vi "sub_SPNs.vi"() -> (0 "SPNs":T1(array[cluster])=[{"SPN"=520192, "Name"="转矩P", "SlotType"=enum."Percent", "Unit"=enum."%", "Value"=variant, "Scaling"=0.4, "LowLmt"=0.0, "HighLmt"=100.0, "Offset"=0.0, "Length"=8, "PGN"=65280, "Comment"="设定转矩的P参数", "LastUpdate"=timestamp(0 s since 1904-01-01)}, {"SPN"=520193, "Name"="转矩I", "SlotType"=enum."Percent", "Unit"=enum."%", "Value"=variant, "Scaling"=0.4, "LowLmt"=0.0, "HighLmt"=100.0, "Offset"=0.0, "Length"=8, "PGN"=65280, "Comment"="设定转矩的I参数", "LastUpdate"=timestamp(0 s since 1904-01-01)}, {"SPN"=520194, "Name"="转矩D", "SlotType"=enum."Percent", "Unit"=enum."%", "Value"=variant, "Scaling"=0.4, "LowLmt"=0.0, "HighLmt"=100.0, "Offset"=0.0, "Length"=8, "PGN"=65280, "Comment"="设定转矩的D参数", "LastUpdate"=timestamp(0 s since 1904-01-01)}, {"SPN"=520195, "Name"="激磁P", "SlotType"=enum."Percent", "Unit"=enum."%", "Value"=variant, "Scaling"=0.4, "LowLmt"=0.0, "HighLmt"=100.0, "Offset"=0.0, "Length"=8, "PGN"=65280, "Comment"="设定激磁的P参数", "LastUpdate"=timestamp(0 s since 1904-01-01)}, {"SPN"=520196, "Name"="激磁I", "SlotType"=enum."Percent", "Unit"=enum."%", "Value"=variant, "Scaling"=0.4, "LowLmt"=0.0, "HighLmt"=100.0, "Offset"=0.0, "Length"=8, "PGN"=65280, "Comment"="设定激磁的I参数", "LastUpdate"=timestamp(0 s since 1904-01-01)}, {"SPN"=520197, "Name"="激磁D", "SlotType"=enum."Percent", "Unit"=enum."%", "Value"=variant, "Scaling"=0.4, "LowLmt"=0.0, "HighLmt"=100.0, "Offset"=0.0, "Length"=8, "PGN"=65280, "Comment"="设定激磁的D参数", "LastUpdate"=timestamp(0 s since 1904-01-01)}, {"SPN"=520198, "Name"="怠速转矩", "SlotType"=enum."Percent", "Unit"=enum."%", "Value"=variant, "Scaling"=0.4, "LowLmt"=0.0, "HighLmt"=100.0, "Offset"=0.0, "Length"=8, "PGN"=65280, "Comment"="", "LastUpdate"=timestamp(0 s since 1904-01-01)}, {"SPN"=520199, "Name"="防滑转矩", "SlotType"=enum."Percent", "Unit"=enum."%", "Value"=variant, "Scaling"=0.4, "LowLmt"=0.0, "HighLmt"=100.0, "Offset"=0.0, "Length"=8, "PGN"=65280, "Comment"="", "LastUpdate"=timestamp(0 s since 1904-01-01)}, {"SPN"=520200, "Name"="滑差", "SlotType"=enum."Number of bytes", "Unit"=enum."1", "Value"=variant, "Scaling"=1.0, "LowLmt"=0.0, "HighLmt"=200.0, "Offset"=0.0, "Length"=8, "PGN"=65280, "Comment"="", "LastUpdate"=timestamp(0 s since 1904-01-01)}, {"SPN"=520201, "Name"="S to RPM", "SlotType"=enum."Velocity, rotational", "Unit"=enum."rpm", "Value"=variant, "Scaling"=0.125, "LowLmt"=0.0, "HighLmt"=8031.875, "Offset"=0.0, "Length"=16, "PGN"=65280, "Comment"="", "LastUpdate"=timestamp(0 s since 1904-01-01)}, {"SPN"=520202, "Name"="弱磁速度", "SlotType"=enum."Velocity, rotational", "Unit"=enum."rpm", "Value"=variant, "Scaling"=0.125, "LowLmt"=0.0, "HighLmt"=8031.875, "Offset"=0.0, "Length"=16, "PGN"=65280, "Comment"="", "LastUpdate"=timestamp(0 s since 1904-01-01)}, {"SPN"=520203, "Name"="D-C限制", "SlotType"=enum."Percent", "Unit"=enum."%", "Value"=variant, "Scaling"=0.4, "LowLmt"=0.0, "HighLmt"=100.0, "Offset"=0.0, "Length"=8, "PGN"=65280, "Comment"="限制控制器的最大驱动电流", "LastUpdate"=timestamp(0 s since 1904-01-01)}, {"SPN"=520204, "Name"="1Delta最大", "SlotType"=enum."Percent", "Unit"=enum."%", "Value"=variant, "Scaling"=0.4, "LowLmt"=0.0, "HighLmt"=100.0, "Offset"=0.0, "Length"=8, "PGN"=65280, "Comment"="限制1倍Delta下的最大功率", "LastUpdate"=timestamp(0 s since 1904-01-01)}, {"SPN"=520205, "Name"="R-C限制", "SlotType"=enum."Percent", "Unit"=enum."%", "Value"=variant, "Scaling"=0.4, "LowLmt"=0.0, "HighLmt"=100.0, "Offset"=0.0, "Length"=8, "PGN"=65280, "Comment"="限制最大回馈电流", "LastUpdate"=timestamp(0 s since 1904-01-01)}, {"SPN"=520206, "Name"="额定转速", "SlotType"=enum."Velocity, rotational", "Unit"=enum."rpm", "Value"=variant, "Scaling"=0.125, "LowLmt"=0.0, "HighLmt"=8031.875, "Offset"=0.0, "Length"=16, "PGN"=65280, "Comment"="", "LastUpdate"=timestamp(0 s since 1904-01-01)}, {"SPN"=520207, "Name"="Delta转速", "SlotType"=enum."Velocity, rotational", "Unit"=enum."rpm", "Value"=variant, "Scaling"=0.125, "LowLmt"=0.0, "HighLmt"=8031.875, "Offset"=0.0, "Length"=16, "PGN"=65280, "Comment"="", "LastUpdate"=timestamp(0 s since 1904-01-01)}, {"SPN"=520208, "Name"="额定最大", "SlotType"=enum."Percent", "Unit"=enum."%", "Value"=variant, "Scaling"=0.4, "LowLmt"=0.0, "HighLmt"=100.0, "Offset"=0.0, "Length"=8, "PGN"=65280, "Comment"="限制额定转速下的最大功率", "LastUpdate"=timestamp(0 s since 1904-01-01)}, {"SPN"=520209, "Name"="2Delta最大", "SlotType"=enum."Percent", "Unit"=enum."%", "Value"=variant, "Scaling"=0.4, "LowLmt"=0.0, "HighLmt"=100.0, "Offset"=0.0, "Length"=8, "PGN"=65280, "Comment"="限制2倍Delta下的最大功率", "LastUpdate"=timestamp(0 s since 1904-01-01)}, {"SPN"=520210, "Name"="4Delta最大", "SlotType"=enum."Percent", "Unit"=enum."%", "Value"=variant, "Scaling"=0.4, "LowLmt"=0.0, "HighLmt"=100.0, "Offset"=0.0, "Length"=8, "PGN"=65280, "Comment"="限制4倍Delta下的最大功率", "LastUpdate"=timestamp(0 s since 1904-01-01)}, {"SPN"=520211, "Name"="8Delta最大", "SlotType"=enum."Percent", "Unit"=enum."%", "Value"=variant, "Scaling"=0.4, "LowLmt"=0.0, "HighLmt"=100.0, "Offset"=0.0, "Length"=8, "PGN"=65280, "Comment"="限制8倍Delta下的最大功率", "LastUpdate"=timestamp(0 s since 1904-01-01)}, {"SPN"=520212, "Name"="ACC Rate", "SlotType"=enum."Time", "Unit"=enum."s", "Value"=variant, "Scaling"=0.1, "LowLmt"=0.0, "HighLmt"=25.0, "Offset"=0.0, "Length"=8, "PGN"=65280, "Comment"="当满踏板的时候,设置转矩从0到最大值的响应时间", "LastUpdate"=timestamp(0 s since 1904-01-01)}, {"SPN"=520213, "Name"="ACC R-Rate", "SlotType"=enum."Time", "Unit"=enum."s", "Value"=variant, "Scaling"=0.1, "LowLmt"=0.0, "HighLmt"=25.0, "Offset"=0.0, "Length"=8, "PGN"=65280, "Comment"="当汽车还在加速的时候,松掉加速踏板后,设置开始减速的时间", "LastUpdate"=timestamp(0 s since 1904-01-01)}, {"SPN"=520214, "Name"="B Rate", "SlotType"=enum."Time", "Unit"=enum."s", "Value"=variant, "Scaling"=0.1, "LowLmt"=0.0, "HighLmt"=25.0, "Offset"=0.0, "Length"=8, "PGN"=65280, "Comment"="当汽车还在行使时,踩下刹车踏板后,设置制动转矩开始的时间", "LastUpdate"=timestamp(0 s since 1904-01-01)}, {"SPN"=520215, "Name"="B R-Rate", "SlotType"=enum."Time", "Unit"=enum."s", "Value"=variant, "Scaling"=0.1, "LowLmt"=0.0, "HighLmt"=25.0, "Offset"=0.0, "Length"=8, "PGN"=65280, "Comment"="当汽车在刹车过程中,松掉刹车踏板后,设置制动转矩释放的时间", "LastUpdate"=timestamp(0 s since 1904-01-01)}, {"SPN"=520216, "Name"="加速Min", "SlotType"=enum."Electrical Voltage", "Unit"=enum."V", "Value"=variant, "Scaling"=0.01, "LowLmt"=0.0, "HighLmt"=642.55, "Offset"=0.0, "Length"=16, "PGN"=65280, "Comment"="设置加速踏板的最小电压", "LastUpdate"=timestamp(0 s since 1904-01-01)}, {"SPN"=520217, "Name"="加速Max", "SlotType"=enum."Electrical Voltage", "Unit"=enum."V", "Value"=variant, "Scaling"=0.01, "LowLmt"=0.0, "HighLmt"=642.55, "Offset"=0.0, "Length"=16, "PGN"=65280, "Comment"="设置加速踏板的最大电压", "LastUpdate"=timestamp(0 s since 1904-01-01)}, {"SPN"=520218, "Name"="刹车Min", "SlotType"=enum."Electrical Voltage", "Unit"=enum."V", "Value"=variant, "Scaling"=0.01, "LowLmt"=0.0, "HighLmt"=642.55, "Offset"=0.0, "Length"=16, "PGN"=65280, "Comment"="设置刹车踏板的最小电压", "LastUpdate"=timestamp(0 s since 1904-01-01)}, {"SPN"=520219, "Name"="加速Map", "SlotType"=enum."Percent", "Unit"=enum."%", "Value"=variant, "Scaling"=0.4, "LowLmt"=0.0, "HighLmt"=100.0, "Offset"=0.0, "Length"=8, "PGN"=65280, "Comment"="设置加速踏板对应的加速曲线", "LastUpdate"=timestamp(0 s since 1904-01-01)}, {"SPN"=520220, "Name"="刹车Max", "SlotType"=enum."Electrical Voltage", "Unit"=enum."V", "Value"=variant, "Scaling"=0.01, "LowLmt"=0.0, "HighLmt"=642.55, "Offset"=0.0, "Length"=16, "PGN"=65280, "Comment"="设置刹车踏板的最大电压", "LastUpdate"=timestamp(0 s since 1904-01-01)}, {"SPN"=520221, "Name"="刹车Map", "SlotType"=enum."Percent", "Unit"=enum."%", "Value"=variant, "Scaling"=0.4, "LowLmt"=0.0, "HighLmt"=100.0, "Offset"=0.0, "Length"=8, "PGN"=65280, "Comment"="设置刹车踏板对应的刹车曲线", "LastUpdate"=timestamp(0 s since 1904-01-01)}, {"SPN"=520256, "Name"="远程加速踏板给定", "SlotType"=enum."Percent", "Unit"=enum."%", "Value"=variant, "Scaling"=0.4, "LowLmt"=0.0, "HighLmt"=100.0, "Offset"=0.0, "Length"=8, "PGN"=65281, "Comment"="远程加速踏板给定值", "LastUpdate"=timestamp(0 s since 1904-01-01)}, {"SPN"=520257, "Name"="远程刹车踏板给定", "SlotType"=enum."Percent", "Unit"=enum."%", "Value"=variant, "Scaling"=0.4, "LowLmt"=0.0, "HighLmt"=100.0, "Offset"=0.0, "Length"=8, "PGN"=65281, "Comment"="远程刹车踏板给定值", "LastUpdate"=timestamp(0 s since 1904-01-01)}, {"SPN"=520258, "Name"="远程档位给定", "SlotType"=enum."Bit Field", "Unit"=enum."1", "Value"=variant, "Scaling"=0.0, "LowLmt"=0.0, "HighLmt"=250.0, "Offset"=0.0, "Length"=8, "PGN"=65281, "Comment"="1:P,2:N,3:D,4:R", "LastUpdate"=timestamp(0 s since 1904-01-01)}, {"SPN"=520259, "Name"="远程调试模式使能", "SlotType"=enum."Bool", "Unit"=enum."bit", "Value"=variant, "Scaling"=0.0, "LowLmt"=0.0, "HighLmt"=1.0, "Offset"=0.0, "Length"=1, "PGN"=65281, "Comment"="远程调试模式开关", "LastUpdate"=timestamp(0 s since 1904-01-01)}, {"SPN"=520260, "Name"="远程加速踏板给定使能", "SlotType"=enum."Bool", "Unit"=enum."bit", "Value"=variant, "Scaling"=0.0, "LowLmt"=0.0, "HighLmt"=1.0, "Offset"=0.0, "Length"=1, "PGN"=65281, "Comment"="远程加速踏板给定开关，远程调试模式开关=T时有效", "LastUpdate"=timestamp(0 s since 1904-01-01)}, {"SPN"=520261, "Name"="远程刹车踏板给定使能", "SlotType"=enum."Bool", "Unit"=enum."bit", "Value"=variant, "Scaling"=0.0, "LowLmt"=0.0, "HighLmt"=1.0, "Offset"=0.0, "Length"=1, "PGN"=65281, "Comment"="远程刹车踏板给定开关，远程调试模式开关=T时有效", "LastUpdate"=timestamp(0 s since 1904-01-01)}, {"SPN"=520262, "Name"="远程档位给定使能", "SlotType"=enum."Bool", "Unit"=enum."bit", "Value"=variant, "Scaling"=0.0, "LowLmt"=0.0, "HighLmt"=1.0, "Offset"=0.0, "Length"=1, "PGN"=65281, "Comment"="远程档位给定开关，远程调试模式开关=T时有效", "LastUpdate"=timestamp(0 s since 1904-01-01)}, {"SPN"=520266, "Name"="给定电压", "SlotType"=enum."Percent", "Unit"=enum."%", "Value"=variant, "Scaling"=0.002, "LowLmt"=0.0, "HighLmt"=100.0, "Offset"=0.0, "Length"=16, "PGN"=65282, "Comment"="压频模式给定电压百分比", "LastUpdate"=timestamp(0 s since 1904-01-01)}, {"SPN"=520267, "Name"="给定频率", "SlotType"=enum."Percent", "Unit"=enum."%", "Value"=variant, "Scaling"=0.002, "LowLmt"=0.0, "HighLmt"=100.0, "Offset"=0.0, "Length"=16, "PGN"=65282, "Comment"="压频模式给定频率百分比", "LastUpdate"=timestamp(0 s since 1904-01-01)}, {"SPN"=520268, "Name"="给定电压使能", "SlotType"=enum."Bool", "Unit"=enum."bit", "Value"=variant, "Scaling"=0.0, "LowLmt"=0.0, "HighLmt"=1.0, "Offset"=0.0, "Length"=1, "PGN"=65282, "Comment"="是否允许通过通信方式给定电压", "LastUpdate"=timestamp(0 s since 1904-01-01)}, {"SPN"=520269, "Name"="给定频率使能", "SlotType"=enum."Bool", "Unit"=enum."bit", "Value"=variant, "Scaling"=0.0, "LowLmt"=0.0, "HighLmt"=1.0, "Offset"=0.0, "Length"=1, "PGN"=65282, "Comment"="是否允许通过通信方式给定频率", "LastUpdate"=timestamp(0 s since 1904-01-01)}, {"SPN"=520272, "Name"="电机转速", "SlotType"=enum."Velocity, rotational", "Unit"=enum."rpm", "Value"=variant, "Scaling"=0.153, "LowLmt"=0.0, "HighLmt"=10000.0, "Offset"=0.0, "Length"=16, "PGN"=65290, "Comment"="电机的转速", "LastUpdate"=timestamp(0 s since 1904-01-01)}, {"SPN"=520273, "Name"="控制器温度", "SlotType"=enum."Temperature", "Unit"=enum."℃", "Value"=variant, "Scaling"=0.03125, "LowLmt"=-273.0, "HighLmt"=1735.0, "Offset"=-273.0, "Length"=16, "PGN"=65290, "Comment"="控制器实际温度", "LastUpdate"=timestamp(0 s since 1904-01-01)}, {"SPN"=520274, "Name"="电机温度", "SlotType"=enum."Temperature", "Unit"=enum."℃", "Value"=variant, "Scaling"=0.03125, "LowLmt"=-273.0, "HighLmt"=1735.0, "Offset"=-273.0, "Length"=16, "PGN"=65290, "Comment"="电机的实际温度", "LastUpdate"=timestamp(0 s since 1904-01-01)}, {"SPN"=520275, "Name"="控制器过压", "SlotType"=enum."Bool", "Unit"=enum."bit", "Value"=variant, "Scaling"=1.0, "LowLmt"=0.0, "HighLmt"=1.0, "Offset"=0.0, "Length"=1, "PGN"=65290, "Comment"="指示控制器是否过压", "LastUpdate"=timestamp(0 s since 1904-01-01)}, {"SPN"=520276, "Name"="控制器欠压", "SlotType"=enum."Bool", "Unit"=enum."bit", "Value"=variant, "Scaling"=1.0, "LowLmt"=0.0, "HighLmt"=1.0, "Offset"=0.0, "Length"=1, "PGN"=65290, "Comment"="指示控制器是否欠压", "LastUpdate"=timestamp(0 s since 1904-01-01)}, {"SPN"=520277, "Name"="控制器过流", "SlotType"=enum."Bool", "Unit"=enum."bit", "Value"=variant, "Scaling"=1.0, "LowLmt"=0.0, "HighLmt"=1.0, "Offset"=0.0, "Length"=1, "PGN"=65290, "Comment"="指示控制器是否过流", "LastUpdate"=timestamp(0 s since 1904-01-01)}, {"SPN"=520278, "Name"="控制器过温", "SlotType"=enum."Bool", "Unit"=enum."bit", "Value"=variant, "Scaling"=1.0, "LowLmt"=0.0, "HighLmt"=1.0, "Offset"=0.0, "Length"=1, "PGN"=65290, "Comment"="指示控制器是否过温", "LastUpdate"=timestamp(0 s since 1904-01-01)}, {"SPN"=520279, "Name"="控制器保护", "SlotType"=enum."Bool", "Unit"=enum."bit", "Value"=variant, "Scaling"=1.0, "LowLmt"=0.0, "HighLmt"=1.0, "Offset"=0.0, "Length"=1, "PGN"=65290, "Comment"="指示控制器是否保护", "LastUpdate"=timestamp(0 s since 1904-01-01)}, {"SPN"=520280, "Name"="其他故障", "SlotType"=enum."Bool", "Unit"=enum."bit", "Value"=variant, "Scaling"=1.0, "LowLmt"=0.0, "HighLmt"=1.0, "Offset"=0.0, "Length"=1, "PGN"=65290, "Comment"="指示控制器是否发生其他故障", "LastUpdate"=timestamp(0 s since 1904-01-01)}, {"SPN"=520281, "Name"="母线电流", "SlotType"=enum."Electrical Current", "Unit"=enum."A", "Value"=variant, "Scaling"=0.05, "LowLmt"=-1600.0, "HighLmt"=1612.75, "Offset"=-1600.0, "Length"=16, "PGN"=65290, "Comment"="电池组母线电流", "LastUpdate"=timestamp(0 s since 1904-01-01)}, {"SPN"=520288, "Name"="母线电压", "SlotType"=enum."Electrical Voltage", "Unit"=enum."V", "Value"=variant, "Scaling"=0.01, "LowLmt"=0.0, "HighLmt"=642.55, "Offset"=0.0, "Length"=16, "PGN"=65291, "Comment"="电池组母线电压", "LastUpdate"=timestamp(0 s since 1904-01-01)}, {"SPN"=520289, "Name"="电机电压", "SlotType"=enum."Electrical Voltage", "Unit"=enum."V", "Value"=variant, "Scaling"=0.01, "LowLmt"=0.0, "HighLmt"=642.55, "Offset"=0.0, "Length"=16, "PGN"=65291, "Comment"="电机端电压有效值", "LastUpdate"=timestamp(0 s since 1904-01-01)}, {"SPN"=520290, "Name"="电机电流", "SlotType"=enum."Electrical Current", "Unit"=enum."A", "Value"=variant, "Scaling"=0.05, "LowLmt"=-1600.0, "HighLmt"=1612.75, "Offset"=-1600.0, "Length"=16, "PGN"=65291, "Comment"="电机端电流有效值", "LastUpdate"=timestamp(0 s since 1904-01-01)}, {"SPN"=520291, "Name"="档位", "SlotType"=enum."Bit Field", "Unit"=enum."1", "Value"=variant, "Scaling"=1.0, "LowLmt"=0.0, "HighLmt"=250.0, "Offset"=0.0, "Length"=4, "PGN"=65291, "Comment"="1:P,2:N,3:D,4:R", "LastUpdate"=timestamp(0 s since 1904-01-01)}, {"SPN"=520292, "Name"="加速给定", "SlotType"=enum."Percent", "Unit"=enum."%", "Value"=variant, "Scaling"=0.4, "LowLmt"=0.0, "HighLmt"=100.0, "Offset"=0.0, "Length"=8, "PGN"=65291, "Comment"="加速踏板百分比", "LastUpdate"=timestamp(0 s since 1904-01-01)}, {"SPN"=520293, "Name"="刹车给定", "SlotType"=enum."Percent", "Unit"=enum."%", "Value"=variant, "Scaling"=0.4, "LowLmt"=0.0, "HighLmt"=100.0, "Offset"=0.0, "Length"=8, "PGN"=65291, "Comment"="刹车踏板百分比", "LastUpdate"=timestamp(0 s since 1904-01-01)}, {"SPN"=520294, "Name"="频率", "SlotType"=enum."Frequency", "Unit"=enum."Hz", "Value"=variant, "Scaling"=0.0078125, "LowLmt"=0.0, "HighLmt"=501.9921875, "Offset"=0.0, "Length"=16, "PGN"=65291, "Comment"="电机同步频率", "LastUpdate"=timestamp(0 s since 1904-01-01)}, {"SPN"=520295, "Name"="直流功率", "SlotType"=enum."Power, Real", "Unit"=enum."kW", "Value"=variant, "Scaling"=0.002, "LowLmt"=0.0, "HighLmt"=128.51, "Offset"=0.0, "Length"=16, "PGN"=65291, "Comment"="控制器直流母线输入功率", "LastUpdate"=timestamp(0 s since 1904-01-01)}, {"SPN"=520296, "Name"="加速开关", "SlotType"=enum."Bool", "Unit"=enum."bit", "Value"=variant, "Scaling"=1.0, "LowLmt"=0.0, "HighLmt"=1.0, "Offset"=0.0, "Length"=1, "PGN"=65291, "Comment"="指示汽车加速踏板是否塌下", "LastUpdate"=timestamp(0 s since 1904-01-01)}, {"SPN"=520297, "Name"="刹车开关", "SlotType"=enum."Bool", "Unit"=enum."bit", "Value"=variant, "Scaling"=1.0, "LowLmt"=0.0, "HighLmt"=1.0, "Offset"=0.0, "Length"=1, "PGN"=65291, "Comment"="指示汽车刹车踏板是否塌下", "LastUpdate"=timestamp(0 s since 1904-01-01)}, {"SPN"=520298, "Name"="座椅开关", "SlotType"=enum."Bool", "Unit"=enum."bit", "Value"=variant, "Scaling"=1.0, "LowLmt"=0.0, "HighLmt"=1.0, "Offset"=0.0, "Length"=1, "PGN"=65291, "Comment"="指示汽车驾驶员座椅是否处于坐姿状态", "LastUpdate"=timestamp(0 s since 1904-01-01)}, {"SPN"=520299, "Name"="电机正转", "SlotType"=enum."Bool", "Unit"=enum."bit", "Value"=variant, "Scaling"=1.0, "LowLmt"=0.0, "HighLmt"=1.0, "Offset"=0.0, "Length"=1, "PGN"=65291, "Comment"="电机正转还是反转", "LastUpdate"=timestamp(0 s since 1904-01-01)}, {"SPN"=520304, "Name"="母线电压", "SlotType"=enum."Electrical Voltage", "Unit"=enum."V", "Value"=variant, "Scaling"=0.01, "LowLmt"=0.0, "HighLmt"=642.55, "Offset"=0.0, "Length"=16, "PGN"=65292, "Comment"="电池组母线电压", "LastUpdate"=timestamp(0 s since 1904-01-01)}, {"SPN"=520305, "Name"="电机电压", "SlotType"=enum."Electrical Voltage", "Unit"=enum."V", "Value"=variant, "Scaling"=0.01, "LowLmt"=0.0, "HighLmt"=642.55, "Offset"=0.0, "Length"=16, "PGN"=65292, "Comment"="电机端电压有效值", "LastUpdate"=timestamp(0 s since 1904-01-01)}, {"SPN"=520306, "Name"="给定电压", "SlotType"=enum."Electrical Voltage", "Unit"=enum."%", "Value"=variant, "Scaling"=0.01, "LowLmt"=0.0, "HighLmt"=642.55, "Offset"=0.0, "Length"=16, "PGN"=65292, "Comment"="给定电压百分比", "LastUpdate"=timestamp(0 s since 1904-01-01)}, {"SPN"=520307, "Name"="效率", "SlotType"=enum."Percent", "Unit"=enum."%", "Value"=variant, "Scaling"=0.4, "LowLmt"=0.0, "HighLmt"=100.0, "Offset"=0.0, "Length"=8, "PGN"=65292, "Comment"="控制器效率", "LastUpdate"=timestamp(0 s since 1904-01-01)}, {"SPN"=520308, "Name"="U相电流", "SlotType"=enum."Electrical Current", "Unit"=enum."A", "Value"=variant, "Scaling"=0.05, "LowLmt"=-1600.0, "HighLmt"=1612.75, "Offset"=-1600.0, "Length"=16, "PGN"=65292, "Comment"="电机U相电流有效值", "LastUpdate"=timestamp(0 s since 1904-01-01)}, {"SPN"=520309, "Name"="V相电流", "SlotType"=enum."Electrical Current", "Unit"=enum."A", "Value"=variant, "Scaling"=0.05, "LowLmt"=-1600.0, "HighLmt"=1612.75, "Offset"=-1600.0, "Length"=16, "PGN"=65292, "Comment"="电机V相电流有效值", "LastUpdate"=timestamp(0 s since 1904-01-01)}, {"SPN"=520310, "Name"="W相电流", "SlotType"=enum."Electrical Current", "Unit"=enum."A", "Value"=variant, "Scaling"=0.05, "LowLmt"=-1600.0, "HighLmt"=1612.75, "Offset"=-1600.0, "Length"=16, "PGN"=65292, "Comment"="电机W相电流有效值", "LastUpdate"=timestamp(0 s since 1904-01-01)}, {"SPN"=520311, "Name"="电机正转", "SlotType"=enum."Bool", "Unit"=enum."bit", "Value"=variant, "Scaling"=1.0, "LowLmt"=0.0, "HighLmt"=1.0, "Offset"=0.0, "Length"=1, "PGN"=65292, "Comment"="电机正转还是反转", "LastUpdate"=timestamp(0 s since 1904-01-01)}, {"SPN"=520312, "Name"="后退", "SlotType"=enum."Bool", "Unit"=enum."bit", "Value"=variant, "Scaling"=1.0, "LowLmt"=0.0, "HighLmt"=1.0, "Offset"=0.0, "Length"=1, "PGN"=65292, "Comment"="是否倒档", "LastUpdate"=timestamp(0 s since 1904-01-01)}, {"SPN"=520313, "Name"="前进", "SlotType"=enum."Bool", "Unit"=enum."bit", "Value"=variant, "Scaling"=1.0, "LowLmt"=0.0, "HighLmt"=1.0, "Offset"=0.0, "Length"=1, "PGN"=65292, "Comment"="是否前进档", "LastUpdate"=timestamp(0 s since 1904-01-01)}, {"SPN"=520314, "Name"="加速踏板", "SlotType"=enum."Bool", "Unit"=enum."bit", "Value"=variant, "Scaling"=1.0, "LowLmt"=0.0, "HighLmt"=1.0, "Offset"=0.0, "Length"=1, "PGN"=65292, "Comment"="加速踏板已踏下", "LastUpdate"=timestamp(0 s since 1904-01-01)}, {"SPN"=520315, "Name"="刹车踏板", "SlotType"=enum."Bool", "Unit"=enum."bit", "Value"=variant, "Scaling"=1.0, "LowLmt"=0.0, "HighLmt"=1.0, "Offset"=0.0, "Length"=1, "PGN"=65292, "Comment"="刹车踏板已踏下", "LastUpdate"=timestamp(0 s since 1904-01-01)}, {"SPN"=520316, "Name"="巡航开关", "SlotType"=enum."Bool", "Unit"=enum."bit", "Value"=variant, "Scaling"=1.0, "LowLmt"=0.0, "HighLmt"=1.0, "Offset"=0.0, "Length"=1, "PGN"=65292, "Comment"="巡航功能开启", "LastUpdate"=timestamp(0 s since 1904-01-01)}, {"SPN"=520317, "Name"="座椅开关", "SlotType"=enum."Bool", "Unit"=enum."bit", "Value"=variant, "Scaling"=1.0, "LowLmt"=0.0, "HighLmt"=1.0, "Offset"=0.0, "Length"=1, "PGN"=65292, "Comment"="座椅开关", "LastUpdate"=timestamp(0 s since 1904-01-01)}, {"SPN"=520318, "Name"="给定频率", "SlotType"=enum."Frequency", "Unit"=enum."Hz", "Value"=variant, "Scaling"=0.0078125, "LowLmt"=0.0, "HighLmt"=501.9921875, "Offset"=0.0, "Length"=16, "PGN"=65292, "Comment"="给定频率值", "LastUpdate"=timestamp(0 s since 1904-01-01)}, {"SPN"=520319, "Name"="频率", "SlotType"=enum."Frequency", "Unit"=enum."Hz", "Value"=variant, "Scaling"=0.0078125, "LowLmt"=0.0, "HighLmt"=501.9921875, "Offset"=0.0, "Length"=16, "PGN"=65292, "Comment"="电机同步频率值", "LastUpdate"=timestamp(0 s since 1904-01-01)}, {"SPN"=520320, "Name"="转差频率", "SlotType"=enum."Frequency", "Unit"=enum."Hz", "Value"=variant, "Scaling"=0.0078125, "LowLmt"=0.0, "HighLmt"=501.9921875, "Offset"=0.0, "Length"=16, "PGN"=65292, "Comment"="转差频率值", "LastUpdate"=timestamp(0 s since 1904-01-01)}, {"SPN"=520321, "Name"="直流功率", "SlotType"=enum."Power, Real", "Unit"=enum."kW", "Value"=variant, "Scaling"=0.002, "LowLmt"=0.0, "HighLmt"=128.51, "Offset"=0.0, "Length"=16, "PGN"=65292, "Comment"="控制器直流母线输入功率", "LastUpdate"=timestamp(0 s since 1904-01-01)}, {"SPN"=520322, "Name"="输出功率", "SlotType"=enum."Power, Real", "Unit"=enum."kW", "Value"=variant, "Scaling"=0.002, "LowLmt"=0.0, "HighLmt"=128.51, "Offset"=0.0, "Length"=16, "PGN"=65292, "Comment"="控制器输出功率", "LastUpdate"=timestamp(0 s since 1904-01-01)}, {"SPN"=520323, "Name"="输出转矩", "SlotType"=enum."Torque", "Unit"=enum."Nm", "Value"=variant, "Scaling"=0.01, "LowLmt"=-320.0, "HighLmt"=322.55, "Offset"=-320.0, "Length"=16, "PGN"=65292, "Comment"="输出转矩值", "LastUpdate"=timestamp(0 s since 1904-01-01)}, {"SPN"=520324, "Name"="给定转速", "SlotType"=enum."Velocity, rotational", "Unit"=enum."rpm", "Value"=variant, "Scaling"=0.125, "LowLmt"=0.0, "HighLmt"=8031.875, "Offset"=0.0, "Length"=16, "PGN"=65292, "Comment"="电机的给定转速", "LastUpdate"=timestamp(0 s since 1904-01-01)}, {"SPN"=520325, "Name"="转差转速", "SlotType"=enum."Velocity, rotational", "Unit"=enum."rpm", "Value"=variant, "Scaling"=0.125, "LowLmt"=0.0, "HighLmt"=8031.875, "Offset"=0.0, "Length"=16, "PGN"=65292, "Comment"="电机的转差转速", "LastUpdate"=timestamp(0 s since 1904-01-01)}, {"SPN"=520326, "Name"="给定电压百分比", "SlotType"=enum."Percent", "Unit"=enum."%", "Value"=variant, "Scaling"=0.01, "LowLmt"=0.0, "HighLmt"=100.0, "Offset"=0.0, "Length"=16, "PGN"=65292, "Comment"="给定电压与母线电压的比值×100%", "LastUpdate"=timestamp(0 s since 1904-01-01)}] {"LastUpdate" format="%<%.3X>T"})   [LabVIEW 2011]
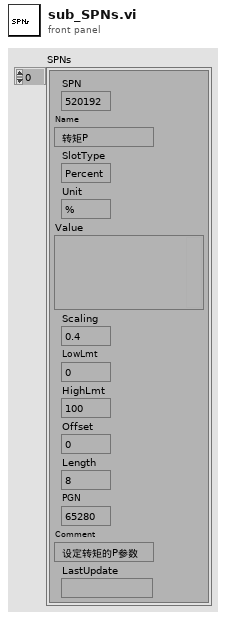
[diagram p1: front panel]
types:
  T1 = cluster{"SPN":u32, "Name":string, "SlotType":enum16{"Unknown Type", "Acceleration", "Angle", "ASCII", "Bool", "Brake Applications", "Bit Field", "Number of bytes", "Capacity, Battery", "Control byte", "Calendar, days", "Calendar, months", "Conductivity", "Count", "Calendar, weeks", "Calendar, years", "Dielectricity", "Direction", "Distance", "Electrical Current", "Economy, gaseous", "Economy, liquid", "Energy", "Electrical Voltage", "Flow rate, gaseous", "Flow rate, liquid", "FMI", "Frequency", "Force", "Fuel Used,gaseous", "Fuel Used, liquid", "Flow rate,volumetric", "Group Function", "Governor gain", "Gear Ratio", "Gear Value", "Identifier", "Inertia", "Intensity, optical", "Kinematic viscosity", "level", "Mass,cargo", "Name (short)", "Name (long)", "OC", "Power, Apparent", "Percent", "Percent,concentration", "Proprietary Data", "position", "Power Factor", "Parts Per Million", "Pressure", "Pressure Rate Change", "Power, Reactive", "Power, Real", "Ratio", "Road Curvature", "Record", "Revolutions", "Source Address", "Specific Gravity", "SPN", "Specific Resistance", "Step", "Transfer Data", "Time", "Temperature", "Torque", "Velocity,angular", "VariantData", "Velocity, linear", "Velocity, magnitude", "Volume", "Velocity, rotational"}, "Unit":enum16{"UnDefined", "%", "1", "1/km", "A", "ASCII", "bin", "bit", "℃", "D", "deg", "deg/s", "g", "Hz", "ID", "kg", "kg/h", "kg/m^2", "km", "km/kg", "km/L", "kPa", "kph", "kW", "kWh", "L", "L/h", "m", "m/h", "m/s", "m/s^2", "m^3/h", "mAh", "min", "mm", "mm^2/s", "Mon", "ms", "mSi/mm", "mW/cm^2", "N", "Nm", "Pa/s", "ppm", "r", "rad/s", "Rat", "Rec", "rpm", "s", "SA", "step", "TF", "V", "VA", "VAr", "W", "Y", "Ωm"}, "Value":variant, "Scaling":dbl, "LowLmt":dbl, "HighLmt":dbl, "Offset":dbl, "Length":u8, "PGN":u32, "Comment":string, "LastUpdate":timestamp}[]
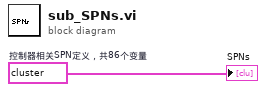
[diagram p0: block diagram]
diagram:
  w1 = T1 [{"SPN"=520192, "Name"="转矩P", "SlotType"=enum."Percent", "Unit"=enum."%", "Value"=variant, "Scaling"=0.4, "LowLmt"=0.0, "HighLmt"=100.0, "Offset"=0.0, "Length"=8, "PGN"=65280, "Comment"="设定转矩的P参数", "LastUpdate"=timestamp(0 s since 1904-01-01)}, {"SPN"=520193, "Name"="转矩I", "SlotType"=enum."Percent", "Unit"=enum."%", "Value"=variant, "Scaling"=0.4, "LowLmt"=0.0, "HighLmt"=100.0, "Offset"=0.0, "Length"=8, "PGN"=65280, "Comment"="设定转矩的I参数", "LastUpdate"=timestamp(0 s since 1904-01-01)}, {"SPN"=520194, "Name"="转矩D", "SlotType"=enum."Percent", "Unit"=enum."%", "Value"=variant, "Scaling"=0.4, "LowLmt"=0.0, "HighLmt"=100.0, "Offset"=0.0, "Length"=8, "PGN"=65280, "Comment"="设定转矩的D参数", "LastUpdate"=timestamp(0 s since 1904-01-01)}, {"SPN"=520195, "Name"="激磁P", "SlotType"=enum."Percent", "Unit"=enum."%", "Value"=variant, "Scaling"=0.4, "LowLmt"=0.0, "HighLmt"=100.0, "Offset"=0.0, "Length"=8, "PGN"=65280, "Comment"="设定激磁的P参数", "LastUpdate"=timestamp(0 s since 1904-01-01)}, {"SPN"=520196, "Name"="激磁I", "SlotType"=enum."Percent", "Unit"=enum."%", "Value"=variant, "Scaling"=0.4, "LowLmt"=0.0, "HighLmt"=100.0, "Offset"=0.0, "Length"=8, "PGN"=65280, "Comment"="设定激磁的I参数", "LastUpdate"=timestamp(0 s since 1904-01-01)}, {"SPN"=520197, "Name"="激磁D", "SlotType"=enum."Percent", "Unit"=enum."%", "Value"=variant, "Scaling"=0.4, "LowLmt"=0.0, "HighLmt"=100.0, "Offset"=0.0, "Length"=8, "PGN"=65280, "Comment"="设定激磁的D参数", "LastUpdate"=timestamp(0 s since 1904-01-01)}, {"SPN"=520198, "Name"="怠速转矩", "SlotType"=enum."Percent", "Unit"=enum."%", "Value"=variant, "Scaling"=0.4, "LowLmt"=0.0, "HighLmt"=100.0, "Offset"=0.0, "Length"=8, "PGN"=65280, "Comment"="", "LastUpdate"=timestamp(0 s since 1904-01-01)}, {"SPN"=520199, "Name"="防滑转矩", "SlotType"=enum."Percent", "Unit"=enum."%", "Value"=variant, "Scaling"=0.4, "LowLmt"=0.0, "HighLmt"=100.0, "Offset"=0.0, "Length"=8, "PGN"=65280, "Comment"="", "LastUpdate"=timestamp(0 s since 1904-01-01)}, {"SPN"=520200, "Name"="滑差", "SlotType"=enum."Number of bytes", "Unit"=enum."1", "Value"=variant, "Scaling"=1.0, "LowLmt"=0.0, "HighLmt"=200.0, "Offset"=0.0, "Length"=8, "PGN"=65280, "Comment"="", "LastUpdate"=timestamp(0 s since 1904-01-01)}, {"SPN"=520201, "Name"="S to RPM", "SlotType"=enum."Velocity, rotational", "Unit"=enum."rpm", "Value"=variant, "Scaling"=0.125, "LowLmt"=0.0, "HighLmt"=8031.875, "Offset"=0.0, "Length"=16, "PGN"=65280, "Comment"="", "LastUpdate"=timestamp(0 s since 1904-01-01)}, {"SPN"=520202, "Name"="弱磁速度", "SlotType"=enum."Velocity, rotational", "Unit"=enum."rpm", "Value"=variant, "Scaling"=0.125, "LowLmt"=0.0, "HighLmt"=8031.875, "Offset"=0.0, "Length"=16, "PGN"=65280, "Comment"="", "LastUpdate"=timestamp(0 s since 1904-01-01)}, {"SPN"=520203, "Name"="D-C限制", "SlotType"=enum."Percent", "Unit"=enum."%", "Value"=variant, "Scaling"=0.4, "LowLmt"=0.0, "HighLmt"=100.0, "Offset"=0.0, "Length"=8, "PGN"=65280, "Comment"="限制控制器的最大驱动电流", "LastUpdate"=timestamp(0 s since 1904-01-01)}, {"SPN"=520204, "Name"="1Delta最大", "SlotType"=enum."Percent", "Unit"=enum."%", "Value"=variant, "Scaling"=0.4, "LowLmt"=0.0, "HighLmt"=100.0, "Offset"=0.0, "Length"=8, "PGN"=65280, "Comment"="限制1倍Delta下的最大功率", "LastUpdate"=timestamp(0 s since 1904-01-01)}, {"SPN"=520205, "Name"="R-C限制", "SlotType"=enum."Percent", "Unit"=enum."%", "Value"=variant, "Scaling"=0.4, "LowLmt"=0.0, "HighLmt"=100.0, "Offset"=0.0, "Length"=8, "PGN"=65280, "Comment"="限制最大回馈电流", "LastUpdate"=timestamp(0 s since 1904-01-01)}, {"SPN"=520206, "Name"="额定转速", "SlotType"=enum."Velocity, rotational", "Unit"=enum."rpm", "Value"=variant, "Scaling"=0.125, "LowLmt"=0.0, "HighLmt"=8031.875, "Offset"=0.0, "Length"=16, "PGN"=65280, "Comment"="", "LastUpdate"=timestamp(0 s since 1904-01-01)}, {"SPN"=520207, "Name"="Delta转速", "SlotType"=enum."Velocity, rotational", "Unit"=enum."rpm", "Value"=variant, "Scaling"=0.125, "LowLmt"=0.0, "HighLmt"=8031.875, "Offset"=0.0, "Length"=16, "PGN"=65280, "Comment"="", "LastUpdate"=timestamp(0 s since 1904-01-01)}, {"SPN"=520208, "Name"="额定最大", "SlotType"=enum."Percent", "Unit"=enum."%", "Value"=variant, "Scaling"=0.4, "LowLmt"=0.0, "HighLmt"=100.0, "Offset"=0.0, "Length"=8, "PGN"=65280, "Comment"="限制额定转速下的最大功率", "LastUpdate"=timestamp(0 s since 1904-01-01)}, {"SPN"=520209, "Name"="2Delta最大", "SlotType"=enum."Percent", "Unit"=enum."%", "Value"=variant, "Scaling"=0.4, "LowLmt"=0.0, "HighLmt"=100.0, "Offset"=0.0, "Length"=8, "PGN"=65280, "Comment"="限制2倍Delta下的最大功率", "LastUpdate"=timestamp(0 s since 1904-01-01)}, {"SPN"=520210, "Name"="4Delta最大", "SlotType"=enum."Percent", "Unit"=enum."%", "Value"=variant, "Scaling"=0.4, "LowLmt"=0.0, "HighLmt"=100.0, "Offset"=0.0, "Length"=8, "PGN"=65280, "Comment"="限制4倍Delta下的最大功率", "LastUpdate"=timestamp(0 s since 1904-01-01)}, {"SPN"=520211, "Name"="8Delta最大", "SlotType"=enum."Percent", "Unit"=enum."%", "Value"=variant, "Scaling"=0.4, "LowLmt"=0.0, "HighLmt"=100.0, "Offset"=0.0, "Length"=8, "PGN"=65280, "Comment"="限制8倍Delta下的最大功率", "LastUpdate"=timestamp(0 s since 1904-01-01)}, {"SPN"=520212, "Name"="ACC Rate", "SlotType"=enum."Time", "Unit"=enum."s", "Value"=variant, "Scaling"=0.1, "LowLmt"=0.0, "HighLmt"=25.0, "Offset"=0.0, "Length"=8, "PGN"=65280, "Comment"="当满踏板的时候,设置转矩从0到最大值的响应时间", "LastUpdate"=timestamp(0 s since 1904-01-01)}, {"SPN"=520213, "Name"="ACC R-Rate", "SlotType"=enum."Time", "Unit"=enum."s", "Value"=variant, "Scaling"=0.1, "LowLmt"=0.0, "HighLmt"=25.0, "Offset"=0.0, "Length"=8, "PGN"=65280, "Comment"="当汽车还在加速的时候,松掉加速踏板后,设置开始减速的时间", "LastUpdate"=timestamp(0 s since 1904-01-01)}, {"SPN"=520214, "Name"="B Rate", "SlotType"=enum."Time", "Unit"=enum."s", "Value"=variant, "Scaling"=0.1, "LowLmt"=0.0, "HighLmt"=25.0, "Offset"=0.0, "Length"=8, "PGN"=65280, "Comment"="当汽车还在行使时,踩下刹车踏板后,设置制动转矩开始的时间", "LastUpdate"=timestamp(0 s since 1904-01-01)}, {"SPN"=520215, "Name"="B R-Rate", "SlotType"=enum."Time", "Unit"=enum."s", "Value"=variant, "Scaling"=0.1, "LowLmt"=0.0, "HighLmt"=25.0, "Offset"=0.0, "Length"=8, "PGN"=65280, "Comment"="当汽车在刹车过程中,松掉刹车踏板后,设置制动转矩释放的时间", "LastUpdate"=timestamp(0 s since 1904-01-01)}, {"SPN"=520216, "Name"="加速Min", "SlotType"=enum."Electrical Voltage", "Unit"=enum."V", "Value"=variant, "Scaling"=0.01, "LowLmt"=0.0, "HighLmt"=642.55, "Offset"=0.0, "Length"=16, "PGN"=65280, "Comment"="设置加速踏板的最小电压", "LastUpdate"=timestamp(0 s since 1904-01-01)}, {"SPN"=520217, "Name"="加速Max", "SlotType"=enum."Electrical Voltage", "Unit"=enum."V", "Value"=variant, "Scaling"=0.01, "LowLmt"=0.0, "HighLmt"=642.55, "Offset"=0.0, "Length"=16, "PGN"=65280, "Comment"="设置加速踏板的最大电压", "LastUpdate"=timestamp(0 s since 1904-01-01)}, {"SPN"=520218, "Name"="刹车Min", "SlotType"=enum."Electrical Voltage", "Unit"=enum."V", "Value"=variant, "Scaling"=0.01, "LowLmt"=0.0, "HighLmt"=642.55, "Offset"=0.0, "Length"=16, "PGN"=65280, "Comment"="设置刹车踏板的最小电压", "LastUpdate"=timestamp(0 s since 1904-01-01)}, {"SPN"=520219, "Name"="加速Map", "SlotType"=enum."Percent", "Unit"=enum."%", "Value"=variant, "Scaling"=0.4, "LowLmt"=0.0, "HighLmt"=100.0, "Offset"=0.0, "Length"=8, "PGN"=65280, "Comment"="设置加速踏板对应的加速曲线", "LastUpdate"=timestamp(0 s since 1904-01-01)}, {"SPN"=520220, "Name"="刹车Max", "SlotType"=enum."Electrical Voltage", "Unit"=enum."V", "Value"=variant, "Scaling"=0.01, "LowLmt"=0.0, "HighLmt"=642.55, "Offset"=0.0, "Length"=16, "PGN"=65280, "Comment"="设置刹车踏板的最大电压", "LastUpdate"=timestamp(0 s since 1904-01-01)}, {"SPN"=520221, "Name"="刹车Map", "SlotType"=enum."Percent", "Unit"=enum."%", "Value"=variant, "Scaling"=0.4, "LowLmt"=0.0, "HighLmt"=100.0, "Offset"=0.0, "Length"=8, "PGN"=65280, "Comment"="设置刹车踏板对应的刹车曲线", "LastUpdate"=timestamp(0 s since 1904-01-01)}, {"SPN"=520256, "Name"="远程加速踏板给定", "SlotType"=enum."Percent", "Unit"=enum."%", "Value"=variant, "Scaling"=0.4, "LowLmt"=0.0, "HighLmt"=100.0, "Offset"=0.0, "Length"=8, "PGN"=65281, "Comment"="远程加速踏板给定值", "LastUpdate"=timestamp(0 s since 1904-01-01)}, {"SPN"=520257, "Name"="远程刹车踏板给定", "SlotType"=enum."Percent", "Unit"=enum."%", "Value"=variant, "Scaling"=0.4, "LowLmt"=0.0, "HighLmt"=100.0, "Offset"=0.0, "Length"=8, "PGN"=65281, "Comment"="远程刹车踏板给定值", "LastUpdate"=timestamp(0 s since 1904-01-01)}, {"SPN"=520258, "Name"="远程档位给定", "SlotType"=enum."Bit Field", "Unit"=enum."1", "Value"=variant, "Scaling"=0.0, "LowLmt"=0.0, "HighLmt"=250.0, "Offset"=0.0, "Length"=8, "PGN"=65281, "Comment"="1:P,2:N,3:D,4:R", "LastUpdate"=timestamp(0 s since 1904-01-01)}, {"SPN"=520259, "Name"="远程调试模式使能", "SlotType"=enum."Bool", "Unit"=enum."bit", "Value"=variant, "Scaling"=0.0, "LowLmt"=0.0, "HighLmt"=1.0, "Offset"=0.0, "Length"=1, "PGN"=65281, "Comment"="远程调试模式开关", "LastUpdate"=timestamp(0 s since 1904-01-01)}, {"SPN"=520260, "Name"="远程加速踏板给定使能", "SlotType"=enum."Bool", "Unit"=enum."bit", "Value"=variant, "Scaling"=0.0, "LowLmt"=0.0, "HighLmt"=1.0, "Offset"=0.0, "Length"=1, "PGN"=65281, "Comment"="远程加速踏板给定开关，远程调试模式开关=T时有效", "LastUpdate"=timestamp(0 s since 1904-01-01)}, {"SPN"=520261, "Name"="远程刹车踏板给定使能", "SlotType"=enum."Bool", "Unit"=enum."bit", "Value"=variant, "Scaling"=0.0, "LowLmt"=0.0, "HighLmt"=1.0, "Offset"=0.0, "Length"=1, "PGN"=65281, "Comment"="远程刹车踏板给定开关，远程调试模式开关=T时有效", "LastUpdate"=timestamp(0 s since 1904-01-01)}, {"SPN"=520262, "Name"="远程档位给定使能", "SlotType"=enum."Bool", "Unit"=enum."bit", "Value"=variant, "Scaling"=0.0, "LowLmt"=0.0, "HighLmt"=1.0, "Offset"=0.0, "Length"=1, "PGN"=65281, "Comment"="远程档位给定开关，远程调试模式开关=T时有效", "LastUpdate"=timestamp(0 s since 1904-01-01)}, {"SPN"=520266, "Name"="给定电压", "SlotType"=enum."Percent", "Unit"=enum."%", "Value"=variant, "Scaling"=0.002, "LowLmt"=0.0, "HighLmt"=100.0, "Offset"=0.0, "Length"=16, "PGN"=65282, "Comment"="压频模式给定电压百分比", "LastUpdate"=timestamp(0 s since 1904-01-01)}, {"SPN"=520267, "Name"="给定频率", "SlotType"=enum."Percent", "Unit"=enum."%", "Value"=variant, "Scaling"=0.002, "LowLmt"=0.0, "HighLmt"=100.0, "Offset"=0.0, "Length"=16, "PGN"=65282, "Comment"="压频模式给定频率百分比", "LastUpdate"=timestamp(0 s since 1904-01-01)}, {"SPN"=520268, "Name"="给定电压使能", "SlotType"=enum."Bool", "Unit"=enum."bit", "Value"=variant, "Scaling"=0.0, "LowLmt"=0.0, "HighLmt"=1.0, "Offset"=0.0, "Length"=1, "PGN"=65282, "Comment"="是否允许通过通信方式给定电压", "LastUpdate"=timestamp(0 s since 1904-01-01)}, {"SPN"=520269, "Name"="给定频率使能", "SlotType"=enum."Bool", "Unit"=enum."bit", "Value"=variant, "Scaling"=0.0, "LowLmt"=0.0, "HighLmt"=1.0, "Offset"=0.0, "Length"=1, "PGN"=65282, "Comment"="是否允许通过通信方式给定频率", "LastUpdate"=timestamp(0 s since 1904-01-01)}, {"SPN"=520272, "Name"="电机转速", "SlotType"=enum."Velocity, rotational", "Unit"=enum."rpm", "Value"=variant, "Scaling"=0.153, "LowLmt"=0.0, "HighLmt"=10000.0, "Offset"=0.0, "Length"=16, "PGN"=65290, "Comment"="电机的转速", "LastUpdate"=timestamp(0 s since 1904-01-01)}, {"SPN"=520273, "Name"="控制器温度", "SlotType"=enum."Temperature", "Unit"=enum."℃", "Value"=variant, "Scaling"=0.03125, "LowLmt"=-273.0, "HighLmt"=1735.0, "Offset"=-273.0, "Length"=16, "PGN"=65290, "Comment"="控制器实际温度", "LastUpdate"=timestamp(0 s since 1904-01-01)}, {"SPN"=520274, "Name"="电机温度", "SlotType"=enum."Temperature", "Unit"=enum."℃", "Value"=variant, "Scaling"=0.03125, "LowLmt"=-273.0, "HighLmt"=1735.0, "Offset"=-273.0, "Length"=16, "PGN"=65290, "Comment"="电机的实际温度", "LastUpdate"=timestamp(0 s since 1904-01-01)}, {"SPN"=520275, "Name"="控制器过压", "SlotType"=enum."Bool", "Unit"=enum."bit", "Value"=variant, "Scaling"=1.0, "LowLmt"=0.0, "HighLmt"=1.0, "Offset"=0.0, "Length"=1, "PGN"=65290, "Comment"="指示控制器是否过压", "LastUpdate"=timestamp(0 s since 1904-01-01)}, {"SPN"=520276, "Name"="控制器欠压", "SlotType"=enum."Bool", "Unit"=enum."bit", "Value"=variant, "Scaling"=1.0, "LowLmt"=0.0, "HighLmt"=1.0, "Offset"=0.0, "Length"=1, "PGN"=65290, "Comment"="指示控制器是否欠压", "LastUpdate"=timestamp(0 s since 1904-01-01)}, {"SPN"=520277, "Name"="控制器过流", "SlotType"=enum."Bool", "Unit"=enum."bit", "Value"=variant, "Scaling"=1.0, "LowLmt"=0.0, "HighLmt"=1.0, "Offset"=0.0, "Length"=1, "PGN"=65290, "Comment"="指示控制器是否过流", "LastUpdate"=timestamp(0 s since 1904-01-01)}, {"SPN"=520278, "Name"="控制器过温", "SlotType"=enum."Bool", "Unit"=enum."bit", "Value"=variant, "Scaling"=1.0, "LowLmt"=0.0, "HighLmt"=1.0, "Offset"=0.0, "Length"=1, "PGN"=65290, "Comment"="指示控制器是否过温", "LastUpdate"=timestamp(0 s since 1904-01-01)}, {"SPN"=520279, "Name"="控制器保护", "SlotType"=enum."Bool", "Unit"=enum."bit", "Value"=variant, "Scaling"=1.0, "LowLmt"=0.0, "HighLmt"=1.0, "Offset"=0.0, "Length"=1, "PGN"=65290, "Comment"="指示控制器是否保护", "LastUpdate"=timestamp(0 s since 1904-01-01)}, {"SPN"=520280, "Name"="其他故障", "SlotType"=enum."Bool", "Unit"=enum."bit", "Value"=variant, "Scaling"=1.0, "LowLmt"=0.0, "HighLmt"=1.0, "Offset"=0.0, "Length"=1, "PGN"=65290, "Comment"="指示控制器是否发生其他故障", "LastUpdate"=timestamp(0 s since 1904-01-01)}, {"SPN"=520281, "Name"="母线电流", "SlotType"=enum."Electrical Current", "Unit"=enum."A", "Value"=variant, "Scaling"=0.05, "LowLmt"=-1600.0, "HighLmt"=1612.75, "Offset"=-1600.0, "Length"=16, "PGN"=65290, "Comment"="电池组母线电流", "LastUpdate"=timestamp(0 s since 1904-01-01)}, {"SPN"=520288, "Name"="母线电压", "SlotType"=enum."Electrical Voltage", "Unit"=enum."V", "Value"=variant, "Scaling"=0.01, "LowLmt"=0.0, "HighLmt"=642.55, "Offset"=0.0, "Length"=16, "PGN"=65291, "Comment"="电池组母线电压", "LastUpdate"=timestamp(0 s since 1904-01-01)}, {"SPN"=520289, "Name"="电机电压", "SlotType"=enum."Electrical Voltage", "Unit"=enum."V", "Value"=variant, "Scaling"=0.01, "LowLmt"=0.0, "HighLmt"=642.55, "Offset"=0.0, "Length"=16, "PGN"=65291, "Comment"="电机端电压有效值", "LastUpdate"=timestamp(0 s since 1904-01-01)}, {"SPN"=520290, "Name"="电机电流", "SlotType"=enum."Electrical Current", "Unit"=enum."A", "Value"=variant, "Scaling"=0.05, "LowLmt"=-1600.0, "HighLmt"=1612.75, "Offset"=-1600.0, "Length"=16, "PGN"=65291, "Comment"="电机端电流有效值", "LastUpdate"=timestamp(0 s since 1904-01-01)}, {"SPN"=520291, "Name"="档位", "SlotType"=enum."Bit Field", "Unit"=enum."1", "Value"=variant, "Scaling"=1.0, "LowLmt"=0.0, "HighLmt"=250.0, "Offset"=0.0, "Length"=4, "PGN"=65291, "Comment"="1:P,2:N,3:D,4:R", "LastUpdate"=timestamp(0 s since 1904-01-01)}, {"SPN"=520292, "Name"="加速给定", "SlotType"=enum."Percent", "Unit"=enum."%", "Value"=variant, "Scaling"=0.4, "LowLmt"=0.0, "HighLmt"=100.0, "Offset"=0.0, "Length"=8, "PGN"=65291, "Comment"="加速踏板百分比", "LastUpdate"=timestamp(0 s since 1904-01-01)}, {"SPN"=520293, "Name"="刹车给定", "SlotType"=enum."Percent", "Unit"=enum."%", "Value"=variant, "Scaling"=0.4, "LowLmt"=0.0, "HighLmt"=100.0, "Offset"=0.0, "Length"=8, "PGN"=65291, "Comment"="刹车踏板百分比", "LastUpdate"=timestamp(0 s since 1904-01-01)}, {"SPN"=520294, "Name"="频率", "SlotType"=enum."Frequency", "Unit"=enum."Hz", "Value"=variant, "Scaling"=0.0078125, "LowLmt"=0.0, "HighLmt"=501.9921875, "Offset"=0.0, "Length"=16, "PGN"=65291, "Comment"="电机同步频率", "LastUpdate"=timestamp(0 s since 1904-01-01)}, {"SPN"=520295, "Name"="直流功率", "SlotType"=enum."Power, Real", "Unit"=enum."kW", "Value"=variant, "Scaling"=0.002, "LowLmt"=0.0, "HighLmt"=128.51, "Offset"=0.0, "Length"=16, "PGN"=65291, "Comment"="控制器直流母线输入功率", "LastUpdate"=timestamp(0 s since 1904-01-01)}, {"SPN"=520296, "Name"="加速开关", "SlotType"=enum."Bool", "Unit"=enum."bit", "Value"=variant, "Scaling"=1.0, "LowLmt"=0.0, "HighLmt"=1.0, "Offset"=0.0, "Length"=1, "PGN"=65291, "Comment"="指示汽车加速踏板是否塌下", "LastUpdate"=timestamp(0 s since 1904-01-01)}, {"SPN"=520297, "Name"="刹车开关", "SlotType"=enum."Bool", "Unit"=enum."bit", "Value"=variant, "Scaling"=1.0, "LowLmt"=0.0, "HighLmt"=1.0, "Offset"=0.0, "Length"=1, "PGN"=65291, "Comment"="指示汽车刹车踏板是否塌下", "LastUpdate"=timestamp(0 s since 1904-01-01)}, {"SPN"=520298, "Name"="座椅开关", "SlotType"=enum."Bool", "Unit"=enum."bit", "Value"=variant, "Scaling"=1.0, "LowLmt"=0.0, "HighLmt"=1.0, "Offset"=0.0, "Length"=1, "PGN"=65291, "Comment"="指示汽车驾驶员座椅是否处于坐姿状态", "LastUpdate"=timestamp(0 s since 1904-01-01)}, {"SPN"=520299, "Name"="电机正转", "SlotType"=enum."Bool", "Unit"=enum."bit", "Value"=variant, "Scaling"=1.0, "LowLmt"=0.0, "HighLmt"=1.0, "Offset"=0.0, "Length"=1, "PGN"=65291, "Comment"="电机正转还是反转", "LastUpdate"=timestamp(0 s since 1904-01-01)}, {"SPN"=520304, "Name"="母线电压", "SlotType"=enum."Electrical Voltage", "Unit"=enum."V", "Value"=variant, "Scaling"=0.01, "LowLmt"=0.0, "HighLmt"=642.55, "Offset"=0.0, "Length"=16, "PGN"=65292, "Comment"="电池组母线电压", "LastUpdate"=timestamp(0 s since 1904-01-01)}, {"SPN"=520305, "Name"="电机电压", "SlotType"=enum."Electrical Voltage", "Unit"=enum."V", "Value"=variant, "Scaling"=0.01, "LowLmt"=0.0, "HighLmt"=642.55, "Offset"=0.0, "Length"=16, "PGN"=65292, "Comment"="电机端电压有效值", "LastUpdate"=timestamp(0 s since 1904-01-01)}, {"SPN"=520306, "Name"="给定电压", "SlotType"=enum."Electrical Voltage", "Unit"=enum."%", "Value"=variant, "Scaling"=0.01, "LowLmt"=0.0, "HighLmt"=642.55, "Offset"=0.0, "Length"=16, "PGN"=65292, "Comment"="给定电压百分比", "LastUpdate"=timestamp(0 s since 1904-01-01)}, {"SPN"=520307, "Name"="效率", "SlotType"=enum."Percent", "Unit"=enum."%", "Value"=variant, "Scaling"=0.4, "LowLmt"=0.0, "HighLmt"=100.0, "Offset"=0.0, "Length"=8, "PGN"=65292, "Comment"="控制器效率", "LastUpdate"=timestamp(0 s since 1904-01-01)}, {"SPN"=520308, "Name"="U相电流", "SlotType"=enum."Electrical Current", "Unit"=enum."A", "Value"=variant, "Scaling"=0.05, "LowLmt"=-1600.0, "HighLmt"=1612.75, "Offset"=-1600.0, "Length"=16, "PGN"=65292, "Comment"="电机U相电流有效值", "LastUpdate"=timestamp(0 s since 1904-01-01)}, {"SPN"=520309, "Name"="V相电流", "SlotType"=enum."Electrical Current", "Unit"=enum."A", "Value"=variant, "Scaling"=0.05, "LowLmt"=-1600.0, "HighLmt"=1612.75, "Offset"=-1600.0, "Length"=16, "PGN"=65292, "Comment"="电机V相电流有效值", "LastUpdate"=timestamp(0 s since 1904-01-01)}, {"SPN"=520310, "Name"="W相电流", "SlotType"=enum."Electrical Current", "Unit"=enum."A", "Value"=variant, "Scaling"=0.05, "LowLmt"=-1600.0, "HighLmt"=1612.75, "Offset"=-1600.0, "Length"=16, "PGN"=65292, "Comment"="电机W相电流有效值", "LastUpdate"=timestamp(0 s since 1904-01-01)}, {"SPN"=520311, "Name"="电机正转", "SlotType"=enum."Bool", "Unit"=enum."bit", "Value"=variant, "Scaling"=1.0, "LowLmt"=0.0, "HighLmt"=1.0, "Offset"=0.0, "Length"=1, "PGN"=65292, "Comment"="电机正转还是反转", "LastUpdate"=timestamp(0 s since 1904-01-01)}, {"SPN"=520312, "Name"="后退", "SlotType"=enum."Bool", "Unit"=enum."bit", "Value"=variant, "Scaling"=1.0, "LowLmt"=0.0, "HighLmt"=1.0, "Offset"=0.0, "Length"=1, "PGN"=65292, "Comment"="是否倒档", "LastUpdate"=timestamp(0 s since 1904-01-01)}, {"SPN"=520313, "Name"="前进", "SlotType"=enum."Bool", "Unit"=enum."bit", "Value"=variant, "Scaling"=1.0, "LowLmt"=0.0, "HighLmt"=1.0, "Offset"=0.0, "Length"=1, "PGN"=65292, "Comment"="是否前进档", "LastUpdate"=timestamp(0 s since 1904-01-01)}, {"SPN"=520314, "Name"="加速踏板", "SlotType"=enum."Bool", "Unit"=enum."bit", "Value"=variant, "Scaling"=1.0, "LowLmt"=0.0, "HighLmt"=1.0, "Offset"=0.0, "Length"=1, "PGN"=65292, "Comment"="加速踏板已踏下", "LastUpdate"=timestamp(0 s since 1904-01-01)}, {"SPN"=520315, "Name"="刹车踏板", "SlotType"=enum."Bool", "Unit"=enum."bit", "Value"=variant, "Scaling"=1.0, "LowLmt"=0.0, "HighLmt"=1.0, "Offset"=0.0, "Length"=1, "PGN"=65292, "Comment"="刹车踏板已踏下", "LastUpdate"=timestamp(0 s since 1904-01-01)}, {"SPN"=520316, "Name"="巡航开关", "SlotType"=enum."Bool", "Unit"=enum."bit", "Value"=variant, "Scaling"=1.0, "LowLmt"=0.0, "HighLmt"=1.0, "Offset"=0.0, "Length"=1, "PGN"=65292, "Comment"="巡航功能开启", "LastUpdate"=timestamp(0 s since 1904-01-01)}, {"SPN"=520317, "Name"="座椅开关", "SlotType"=enum."Bool", "Unit"=enum."bit", "Value"=variant, "Scaling"=1.0, "LowLmt"=0.0, "HighLmt"=1.0, "Offset"=0.0, "Length"=1, "PGN"=65292, "Comment"="座椅开关", "LastUpdate"=timestamp(0 s since 1904-01-01)}, {"SPN"=520318, "Name"="给定频率", "SlotType"=enum."Frequency", "Unit"=enum."Hz", "Value"=variant, "Scaling"=0.0078125, "LowLmt"=0.0, "HighLmt"=501.9921875, "Offset"=0.0, "Length"=16, "PGN"=65292, "Comment"="给定频率值", "LastUpdate"=timestamp(0 s since 1904-01-01)}, {"SPN"=520319, "Name"="频率", "SlotType"=enum."Frequency", "Unit"=enum."Hz", "Value"=variant, "Scaling"=0.0078125, "LowLmt"=0.0, "HighLmt"=501.9921875, "Offset"=0.0, "Length"=16, "PGN"=65292, "Comment"="电机同步频率值", "LastUpdate"=timestamp(0 s since 1904-01-01)}, {"SPN"=520320, "Name"="转差频率", "SlotType"=enum."Frequency", "Unit"=enum."Hz", "Value"=variant, "Scaling"=0.0078125, "LowLmt"=0.0, "HighLmt"=501.9921875, "Offset"=0.0, "Length"=16, "PGN"=65292, "Comment"="转差频率值", "LastUpdate"=timestamp(0 s since 1904-01-01)}, {"SPN"=520321, "Name"="直流功率", "SlotType"=enum."Power, Real", "Unit"=enum."kW", "Value"=variant, "Scaling"=0.002, "LowLmt"=0.0, "HighLmt"=128.51, "Offset"=0.0, "Length"=16, "PGN"=65292, "Comment"="控制器直流母线输入功率", "LastUpdate"=timestamp(0 s since 1904-01-01)}, {"SPN"=520322, "Name"="输出功率", "SlotType"=enum."Power, Real", "Unit"=enum."kW", "Value"=variant, "Scaling"=0.002, "LowLmt"=0.0, "HighLmt"=128.51, "Offset"=0.0, "Length"=16, "PGN"=65292, "Comment"="控制器输出功率", "LastUpdate"=timestamp(0 s since 1904-01-01)}, {"SPN"=520323, "Name"="输出转矩", "SlotType"=enum."Torque", "Unit"=enum."Nm", "Value"=variant, "Scaling"=0.01, "LowLmt"=-320.0, "HighLmt"=322.55, "Offset"=-320.0, "Length"=16, "PGN"=65292, "Comment"="输出转矩值", "LastUpdate"=timestamp(0 s since 1904-01-01)}, {"SPN"=520324, "Name"="给定转速", "SlotType"=enum."Velocity, rotational", "Unit"=enum."rpm", "Value"=variant, "Scaling"=0.125, "LowLmt"=0.0, "HighLmt"=8031.875, "Offset"=0.0, "Length"=16, "PGN"=65292, "Comment"="电机的给定转速", "LastUpdate"=timestamp(0 s since 1904-01-01)}, {"SPN"=520325, "Name"="转差转速", "SlotType"=enum."Velocity, rotational", "Unit"=enum."rpm", "Value"=variant, "Scaling"=0.125, "LowLmt"=0.0, "HighLmt"=8031.875, "Offset"=0.0, "Length"=16, "PGN"=65292, "Comment"="电机的转差转速", "LastUpdate"=timestamp(0 s since 1904-01-01)}, {"SPN"=520326, "Name"="给定电压百分比", "SlotType"=enum."Percent", "Unit"=enum."%", "Value"=variant, "Scaling"=0.01, "LowLmt"=0.0, "HighLmt"=100.0, "Offset"=0.0, "Length"=16, "PGN"=65292, "Comment"="给定电压与母线电压的比值×100%", "LastUpdate"=timestamp(0 s since 1904-01-01)}]  # 控制器相关SPN定义，共86个变量
  "SPNs" <- w1
